vi "Write_PanelBounds.vi"(1 "refnum in":T1, 2 "path":path) -> (0 "refnum out":T1)   [LabVIEW 2011]
uses:
  <vilib>/Utility/config.llb/Config Data RefNum.ctl
  <vilib>/Utility/config.llb/Write Key (I32).vi
  <vilib>/Utility/config.llb/NI_LVConfig.lvlib
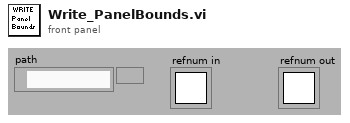
[diagram p1: front panel]
types:
  T1 = typedef "NI_LVConfig.lvlib/Config Data RefNum.ctl" = refnum<k1>
  T2 = typedef "LVRectTypeDef.ctl" = cluster{"left":i16, "top":i16, "right":i16, "bottom":i16}
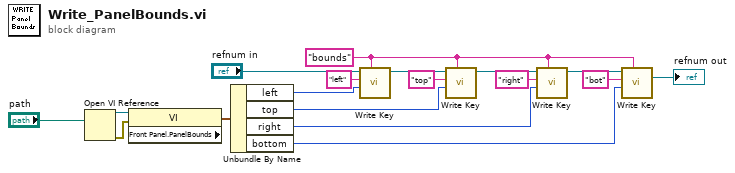
[diagram p0: block diagram]
diagram:
  w13 = "bounds" ("section")
  n1 = Open VI Reference(vi path="path") -> (vi reference=w3:refnum<vi>, error out=w2:errorcluster)  [unwired: 5 in]
  n2 = property class="VI"(reference=w3, error in=w2) -> ("Front Panel.PanelBounds"=w4:T2)  [unwired: 2 out]
  n3 = Unbundle By Name(w4) -> ("left"=w5:i16, "top"=w14:i16, "right"=w15:i16, "bottom"=w16:i16)
  n4 = call-poly <vilib>:"Write Key.vi"("section"=w13, "value"=w5, "key"="left", "refnum"="refnum in") -> ("refnum out"=w12:T1)  [unwired: 5 in, 2 out]
  n5 = call-poly <vilib>:"Write Key.vi"("section"=w13, "value"=w14, "key"="top", "refnum"=w12) -> ("refnum out"=w10:T1)  [unwired: 5 in, 2 out]
  n6 = call-poly <vilib>:"Write Key.vi"("section"=w13, "value"=w15, "key"="right", "refnum"=w10) -> ("refnum out"=w9:T1)  [unwired: 5 in, 2 out]
  n7 = call-poly <vilib>:"Write Key.vi"("section"=w13, "value"=w16, "key"="bot", "refnum"=w9) -> ("refnum out"=→"refnum out":T1)  [unwired: 5 in, 2 out]
